vi "Ball Screw Control.vi"() -> ()   [LabVIEW 2012]
uses:
  Robot Global Data.vi
  <vilib>/Rock Robotics/WPI/CAN/Jaguar/SubVIs/WPI_CANJaguar_ControlMode.ctl
  <vilib>/Rock Robotics/WPI/CAN/Jaguar/SubVIs/WPI_CANJaguar_PositionReference.ctl
  <vilib>/Rock Robotics/WPI/PWM/WPI_PWMTransform_ConPane.ctl
  <vilib>/Rock Robotics/SystemInterfaces/Typedef/FPGA_TypedefDigitalModule.ctl
  <vilib>/Rock Robotics/SystemInterfaces/DIO/FPGA_DIOPWMChannel.ctl
  <vilib>/Rock Robotics/WPI/PWM/WPI_PWMDeadband.ctl
  <vilib>/Rock Robotics/WPI/MotorControl/WPI_MotorControlDeviceRef.ctl
panel:
  in  "Ball Screw DevRef In":T1={"DeviceStatus"={"status"=FALSE, "code"=0, "source"=""}, "Type"=enum."PWM", "PWM"={"Digital Module"=enum."Digital Module 1", "PWM Channel"=enum."Invalid", "DeadBand"={"Name"="", "maxPositivePwm"=0, "minPositivePwm"=0, "centerPwm"=0, "maxNegativePwm"=0, "minNegativePwm"=0, "angularRange"=0}}, "CAN"={"Device Number"=0, "Control Mode"=enum."Percent VBus", "Semaphore"=refnum, "Max Vout"=12.0}, "Invert"=FALSE, "TransformRef"=refnum, "InvTransformRef"=refnum}
  in  "Closed Loop On/Off":bool
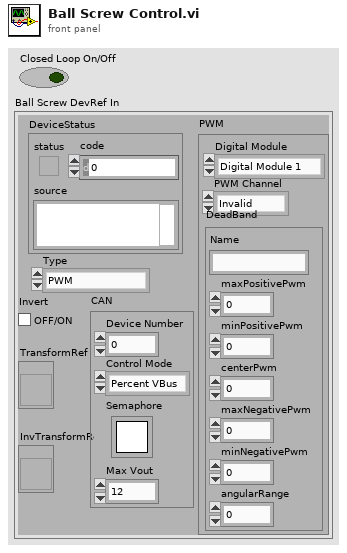
[diagram p1: front panel]
types:
  T1 = typedef "WPI_MotorControlDeviceRef.ctl" = cluster{"DeviceStatus":errorcluster, "Type":enum16{"PWM", "CAN"}, "PWM":cluster{"Digital Module":T2, "PWM Channel":T3, "DeadBand":T4}, "CAN":cluster{"Device Number":u8, "Control Mode":T5, "Semaphore":T6, "Max Vout":dbl}, "Invert":bool, "TransformRef":T7, "InvTransformRef":T7}
  T2 = typedef "FPGA_TypedefDigitalModule.ctl" = enum16{"Digital Module 1", "Digital Module 2"}
  T3 = typedef "FPGA_DIOPWMChannel.ctl" = enum8{"PWM 1", "PWM 2", "PWM 3", "PWM 4", "PWM 5", "PWM 6", "PWM 7", "PWM 8", "PWM 9", "PWM 10", "Invalid"}
  T4 = typedef "WPI_PWMDeadband.ctl" = cluster{"Name":string, "maxPositivePwm":i32, "minPositivePwm":i32, "centerPwm":i32, "maxNegativePwm":i32, "minNegativePwm":i32, "angularRange":u16}
  T5 = typedef "WPI_CANJaguar_ControlMode.ctl" = enum8{"Percent VBus", "Current", "Speed", "Position", "Voltage"}
  T6 = typedef "Semaphore RefNum" = refnum<k1>
  T7 = typedef "WPI_PWMTransform_ConPane.ctl" = refnum<vi>
  T8 = typedef "WPI_CANJaguar_PositionReference.ctl" = u8
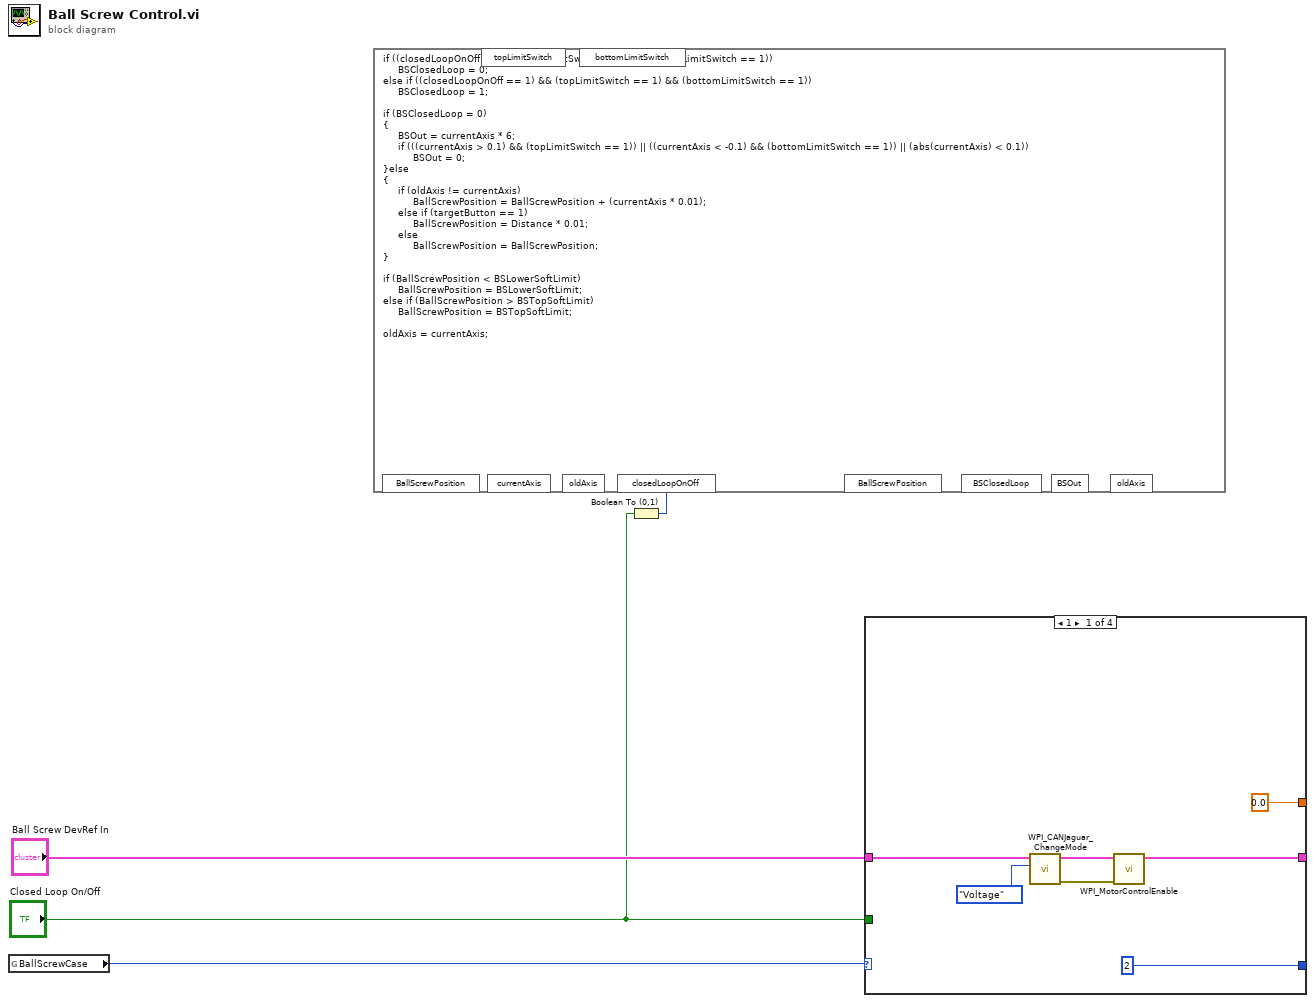
[diagram p0: block diagram]
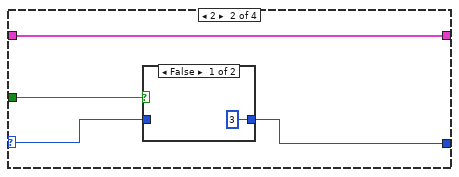
[diagram p2: hidden frame]
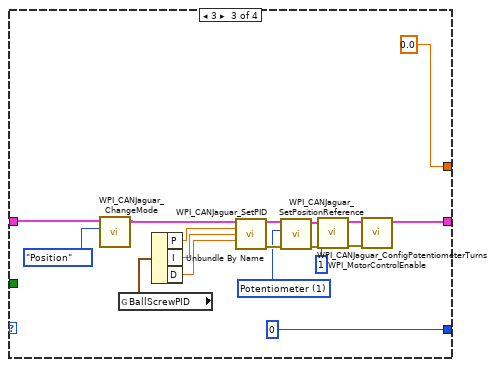
[diagram p4: hidden frame]
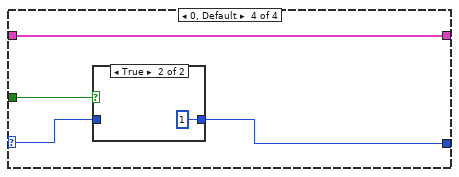
[diagram p5: hidden frame]
diagram:
  n1 = global read "Robot Global Data.vi" "BallScrewCase"() -> (w4:i8)
  n2 = Boolean To (0,1)(Boolean="Closed Loop On/Off") -> (0, 1=w1:i16)
  n3 = formula code="if ((closedLoopOnOff == 1) || (topLimitSwitch == 1) || (bottomLimitSwitch == 1))\n     BSClosedLoop = 0;\nelse if ((closedLoopOnOff == 1) && (topLimitSwitch == 1) && (bottomLimitSwitch == 1))\n     BSClosedLoop = 1;\n\nif (BSClosedLoop = 0)\n{\n     BSOut = currentAxis * 6;\n     if (((currentAxis > 0.1) && (topLimitSwitch == 1)) || ((currentAxis < -0.1) && (bottomLimitSwitch == 1)) || (abs(currentAxis) < 0.1))\n          BSOut = 0;\n}else\n{\n     if (oldAxis != currentAxis)\n          BallScrewPosition = BallScrewPosition + (currentAxis * 0.01);\n     else if (targetButton == 1)\n          BallScrewPosition = Distance * 0.01;\n     else\n          BallScrewPosition = BallScrewPosition;\n}\n\nif (BallScrewPosition < BSLowerSoftLimit)\n     BallScrewPosition = BSLowerSoftLimit;\nelse if (BallScrewPosition > BSTopSoftLimit)\n     BallScrewPosition = BSTopSoftLimit;\n\noldAxis = currentAxis;"("closedLoopOnOff"=w1) -> ()  [unwired: 5 in, 4 out]
  n4 = case shown="1" w4 {
    selector: w4 -> [_ w13 _ w36]
    tunnel: [i8 2 ("ShooterCase") w12 i8 0 ("ShooterCase") w37] -> _
    tunnel: "Ball Screw DevRef In" -> [w10 w15 w34 w39]
    tunnel: [w6 w15 w21 w39] -> _
    tunnel: "Closed Loop On/Off" -> [_ w14 _ w38]
    tunnel: [0.0 ("FSpeed") _ 0.0 ("FSpeed") _] -> _
    frame 1 {
      n5 = call <vilib>:"WPI_CANJaguar_ChangeMode.vi"("Control Mode"=WPI_CANJaguar_ControlMode."Voltage", "CAN Jaguar Ref"=w10) -> ("error out"=w7:errorcluster, "CAN Jaguar Ref Out"=w8:T1)  [unwired: 8 in]
      n6 = call <vilib>:"WPI_MotorControlEnable.vi"("error in (no error)"=w7, "CAN Jaguar Ref"=w8) -> ("CAN Jaguar Ref Out"=w6:T1)  [unwired: 8 in, 1 out]
    }
    frame 2 {
      n7 = case shown="False" w14 {
        tunnel: [i8 3 ("ShooterCase") w17] -> w12
        tunnel: w13 -> [_ w17]
        frame False {
        }
        frame True {
        }
      }
    }
    frame 3 {
      w19 = T8 1 items=["Quad Encoder"=0, "Potentiometer"=1, "None"=255] ("Position Reference")
      n8 = call <vilib>:"WPI_CANJaguar_ChangeMode.vi"("Control Mode"=WPI_CANJaguar_ControlMode."Position", "CAN Jaguar Ref"=w34) -> ("CAN Jaguar Ref Out"=w29:T1)  [unwired: 8 in, 1 out]
      n9 = global read "Robot Global Data.vi" "BallScrewPID"() -> (w33:cluster{"P":dbl, "I":dbl, "D":dbl})
      n10 = Unbundle By Name(w33) -> ("P"=w32:dbl, "I"=w31:dbl, "D"=w30:dbl)
      n11 = call <vilib>:"WPI_CANJaguar_SetPID.vi"("CAN Jaguar Ref"=w29, "P"=w32, "I"=w31, "D"=w30) -> ("CAN Jaguar Ref Out"=w27:T1, "error out"=w26:errorcluster)  [unwired: 10 in]
      n12 = call <vilib>:"WPI_CANJaguar_SetPositionReference.vi"("error in (no error)"=w26, "Position Reference"=w19, "CAN Jaguar Ref"=w27) -> ("error out"=w24:errorcluster, "CAN Jaguar Ref Out"=w25:T1)  [unwired: 7 in]
      n13 = call <vilib>:"WPI_CANJaguar_ConfigPotentiometerTurns.vi"("error in (no error)"=w24, "Potentiometer Turns"=u16 1, "CAN Jaguar Ref"=w25) -> ("error out"=w23:errorcluster, "CAN Jaguar Ref Out"=w22:T1)  [unwired: 7 in]
      n14 = call <vilib>:"WPI_MotorControlEnable.vi"("error in (no error)"=w23, "CAN Jaguar Ref"=w22) -> ("CAN Jaguar Ref Out"=w21:T1)  [unwired: 8 in, 1 out]
    }
    frame 0, Default {
      n15 = case shown="True" w38 {
        tunnel: [w40 i8 1 ("ShooterCase")] -> w37
        tunnel: w36 -> [w40 _]
        frame False {
        }
        frame True {
        }
      }
    }
  }
